vi "Create Process.vi"(8 "error in (no error)":errorcluster, 10 "Sequence":string[](array[string]), 11 "Process Model in":refnum<class "Process Model.lvclass">) -> (0 "error out":errorcluster, 3 "Process Model out":refnum<class "Process Model.lvclass">)   [LabVIEW 2019, in "Process Model.lvclass"]
uses:
  <vilib>/gpm_packages/@cs/Car-wash/Source/Process Model/Process Model.lvclass
  <vilib>/gpm_packages/@cs/test-executive/Source/Test Executive/TestExecutive/Test Executive.lvclass
  C:/Program Files/National Instruments/LabVIEW 2019/vi.lib/gpm_packages/@cs/test-executive/Source/Test Executive/ITestExecutive/ITest Executive.lvclass
  <vilib>/gpm_packages/@cs/Car-wash/Source/Process Model/Process Model.lvclass/Process Model.ctl
  <vilib>/gpm_packages/@cs/test-executive/Source/Test Executive/TestExecutive Ref/TestExecutive Ref.lvclass
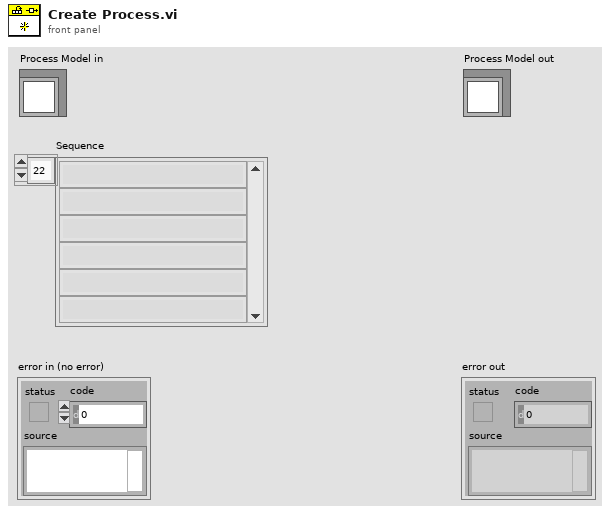
[diagram p1: front panel]
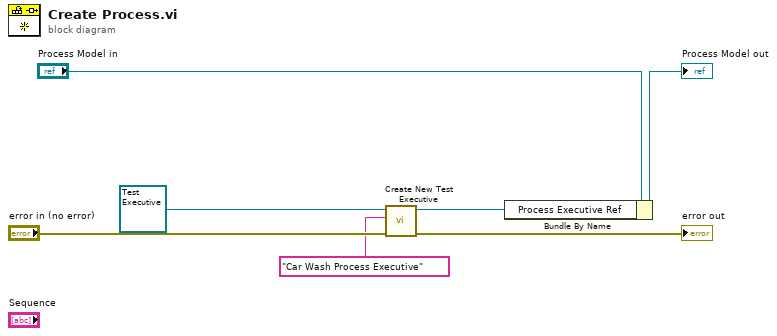
[diagram p0: block diagram]
diagram:
  n1 = call <vilib>:"Create New Test Executive.vi"("error in (no error)"="error in (no error)", "Name"="Car Wash Process Executive", "Test Executive"=refnum<class "Test Executive.lvclass"> refnum ("Test Executive.lvlib:Test Executive.lvclass")) -> ("error out"=→"error out":errorcluster, "Test Executive Ref"=w2:refnum<data-value>)  [unwired: 6 in, 1 out]
  n2 = Bundle By Name(cluster="Process Model in", "Process Executive Ref"=w2) -> (→"Process Model out":refnum<class "Process Model.lvclass">)
